vi "TestComplete.vi"(8 "error in (no error)":errorcluster, 10 "Done":bool, 11 "UnitTestEngine in":refnum<class "UnitTestEngine.lvclass">) -> (0 "error out":errorcluster, 3 "UnitTestEngine out":refnum<class "UnitTestEngine.lvclass">)   [LabVIEW 2019, in "UnitTestEngine.lvlib" / "UnitTestEngine.lvclass"]
uses:
  UnitTestEngine.lvclass
  C:/Program Files (x86)/National Instruments/LabVIEW 2019/vi.lib/NI/Event Source Actor/Event Source/Event Source/Event Source.lvclass
  TestEngine/TestEngine/TestResultInformation.lvclass
  C:/Program Files (x86)/National Instruments/LabVIEW 2019/vi.lib/NI/Event Source Actor/Event Source/Event/Event.lvclass
  <vilib>/NI/Event Source Actor/Event Source/Event/Event.lvclass/Event.ctl
  UnitTestEngine.lvclass/UnitTestEngine.ctl
  <vilib>/NI/Event Source Actor/Event Source/Event/Event.lvclass
  <vilib>/NI/Event Source Actor/Event Source/Event Source/Event Source.lvclass
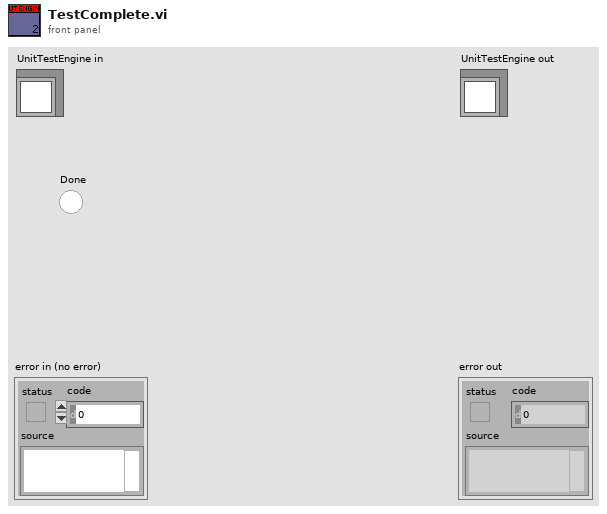
[diagram p1: front panel]
types:
  T1 = cluster{"Text.Text":string, dbl, bool, "Value":string, i32}
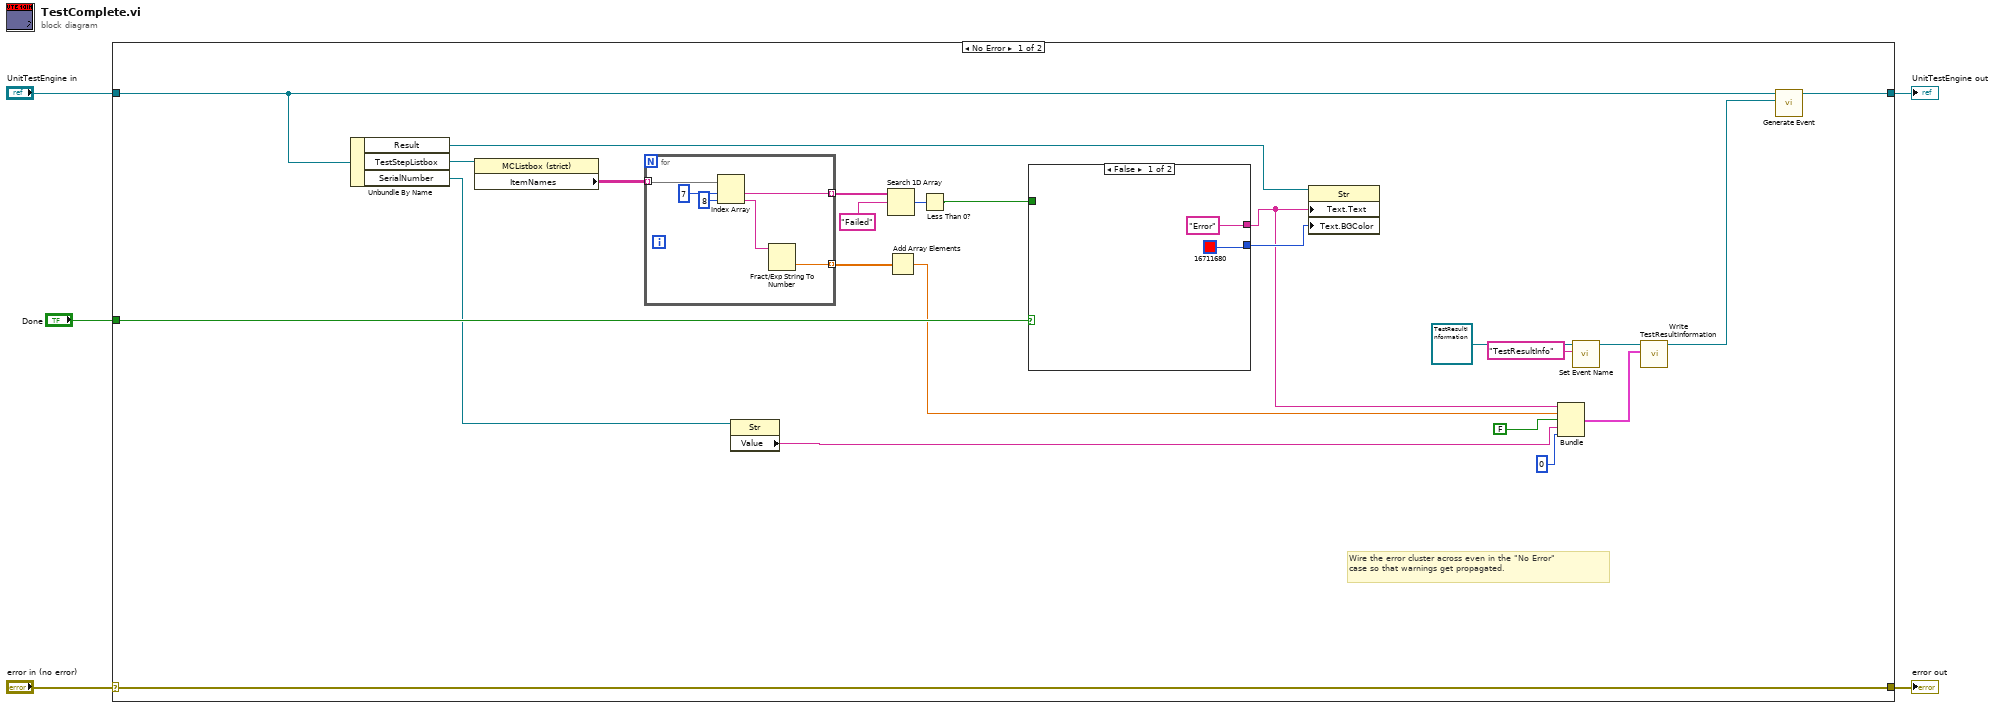
[diagram p0: block diagram]
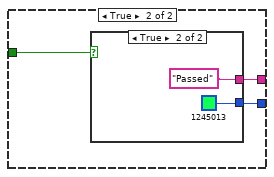
[diagram p2: hidden frame]
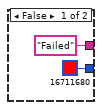
[diagram p3: hidden frame]
diagram:
  n1 = case shown="No Error" "error in (no error)" {
    selector: "error in (no error)" -> [w6 w46]
    tunnel: [w6 w46] -> w4
    tunnel: [w13 w45] -> w2
    tunnel: "UnitTestEngine in" -> [w14 w45]
    tunnel: "Done" -> [w28 _]
    frame No Error {
      # "Wire the error cluster across even in the \"No Error\"\ncase so that warnings get propagated."
      n2 = Unbundle By Name(w14) -> ("Result"=w29:refnum<vi>, "TestStepListbox"=w26:refnum<vi>, "SerialNumber"=w17:refnum<vi>)
      n3 = property class="MCListbox (strict)"(reference=w26) -> ("ItemNames"=w25:string[][])  [unwired: 1 in, 2 out]
      n4 = for {
        tunnel: w25 -> [w35] mode=indexing
        tunnel: [w31] -> w19 mode=indexing
        tunnel: [w30] -> w11 mode=indexing
        n5 = Index Array(array=w35, index #1=7 ("index"), index #2=8 ("index")) -> (element #1=w30:string, element #2=w32:string)
        n6 = Fract/Exp String To Number(string=w32) -> (number=w31:dbl)  [unwired: 3 in, 1 out]
      }
      n7 = property class="Str"(reference=w17) -> ("Value"=w16:string)  [unwired: 1 in, 2 out]
      n8 = Search 1D Array(1D array=w11, element="Failed" ("Text.Text")) -> (index of element=w9:i32)  [unwired: 1 in]
      n9 = Add Array Elements(numeric array=w19) -> (sum=w15:dbl)
      n10 = Less Than 0?(x=w9) -> (x < 0?=w8:bool)
      n11 = case shown="False" w28 {
        tunnel: ["Error" ("Text.Text") w40] -> w20
        tunnel: [u32 16711680 ("Text.Text Colors:Text Color") w39] -> w27
        tunnel: w8 -> [_ w38]
        frame False {
        }
        frame True {
          n12 = case shown="True" w38 {
            tunnel: ["Failed" ("Text.Text") "Passed" ("Text.Text")] -> w40
            tunnel: [u32 16711680 ("Text.Text Colors:Text Color") u32 1245013 ("Text.Text Colors:Text Color")] -> w39
            frame False {
            }
            frame True {
            }
          }
        }
      }
      n13 = property class="Str"(reference=w29, "Text.Text"=w20, "Text.BGColor"=w27) -> ()  [unwired: 1 in, 2 out]
      n14 = Bundle("Text.Text"=w20, w15, FALSE, "Value"=w16, 0) -> (w21:T1)  [unwired: 1 in]
      n15 = call <vilib>:"Set Event Name.vi"("Name (Generic)"="TestResultInfo", "Event In"=refnum<class "TestResultInformation.lvclass"> refnum ("TestEngine.lvlib:TestResultInformation.lvclass")) -> ("Event Out"=w22:refnum<class "TestResultInformation.lvclass">)  [unwired: 9 in]
      n16 = call-dynamic "Write TestResultInformation.vi"("TestResultInformation"=w21, "TestResultInformation in"=w22) -> ("TestResultInformation out"=w12:refnum<class "TestResultInformation.lvclass">)  [unwired: 8 in, 1 out]
      n17 = call <vilib>:"Generate Event.vi"("Event"=w12, "Event Source In"=w14) -> ("Event Source Out"=w13:refnum<class "UnitTestEngine.lvclass">)  [unwired: 8 in, 1 out]
    }
    frame Error {
    }
  }
  "error out" <- w4
  "UnitTestEngine out" <- w2
